vi "ActorDatabase-PerformInsertInstruction.vi"(7 "Payload From Actor":string, 8 "error in (no error)":errorcluster, 11 "Database-Actor in":refnum<class "PartCertDatabase-Actor.lvclass">) -> (0 "error out":errorcluster, 3 "Database-Actor out":refnum<class "PartCertDatabase-Actor.lvclass">)   [LabVIEW 2013, in "PartCertDatabase-Actor.lvclass"]
uses:
  PartCertDatabase-Actor.lvclass
  PartCertDatabase-Actor.lvclass/PartCertDatabase-Actor.ctl
  Reuse Library/Database API/PartCertDatabase-API.lvclass
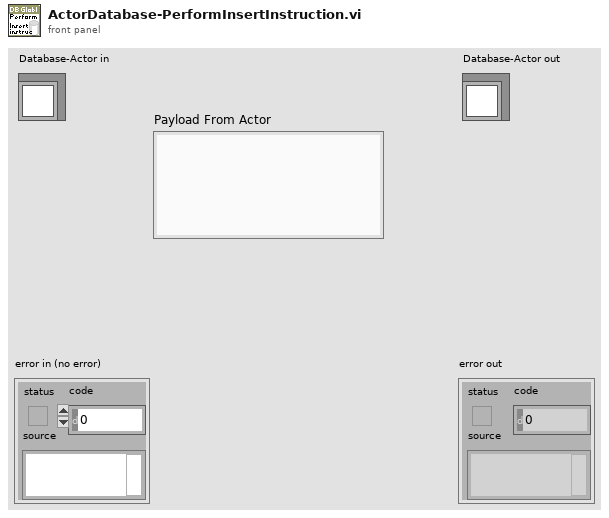
[diagram p1: front panel]
types:
  T1 = cluster{"Table":string, "SQL Statement":string, "Update All":bool, "Payload":string, "Reply Command":string, "Type Of Insertion":i32}
  T2 = cluster{"Manufacturing-Part Number":string, "Step Number":string, "Label Instructions":string, "Path for Picture Label":path, "Path for Picture Label 2":path, "Path for Picture Label 3":path, "Path for Picture Label 4":path, "Path for Picture Label 5":path, "Path for Picture Label 6":path, "Path for Picture Label 7":path, "General Instruction Name":string}[]
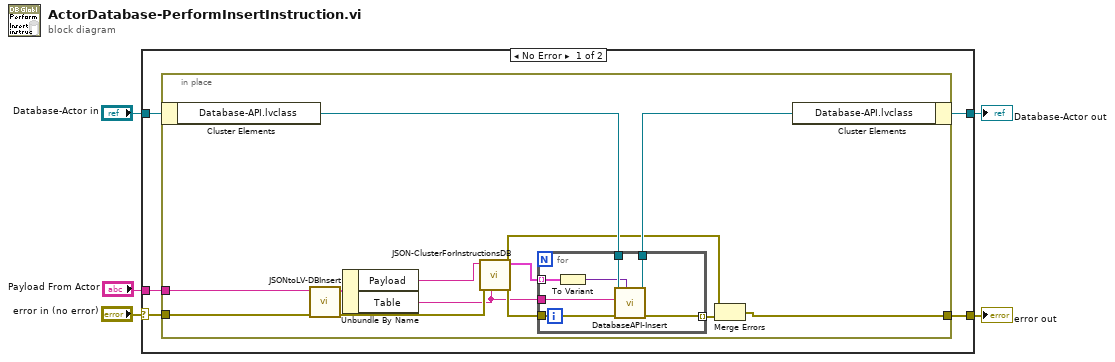
[diagram p0: block diagram]
diagram:
  n1 = case shown="No Error" "error in (no error)" {
    selector: "error in (no error)" -> [w10 w31]
    tunnel: [w9 w31] -> w4
    tunnel: [w7 w30] -> w2
    tunnel: "Database-Actor in" -> [w8 w30]
    tunnel: "Payload From Actor" -> [w6 _]
    frame No Error {
      n2 = in-place {
        in-place-border: w10 -> [w20]
        in-place-border: [w13] -> w9
        in-place-border: w6 -> [w11]
        n3 = in-place-cluster #1(w8) -> ("Database-API.lvclass"=w22:refnum<class "PartCertDatabase-API.lvclass">)
        n4 = call "JSONtoLV-DBInsert.vi"("error in"=w20, "Output JSON Object"=w11) -> ("error out"=w17:errorcluster, "value"=w19:T1)  [unwired: 8 in]
        n5 = Unbundle By Name(w19) -> ("Payload"=w18:string, "Table"=w12:string)
        n6 = call "JSON-ClusterForInstructionsDB.vi"("Table"=w12, "error in (no error)"=w17, "Payload"=w18) -> ("error out"=w14:errorcluster, "Cluster Out"=w16:T2)  [unwired: 7 in]
        n7 = for {
          tunnel: w22 -> [w29]
          tunnel: [w28] -> w21
          tunnel: w12 -> [w27]
          tunnel: w14 -> [w26]
          tunnel: [w25] -> w15 mode=indexing
          tunnel: w16 -> [w24] mode=indexing
          n8 = To Variant(anything=w24) -> (Variant=w23:variant)
          n9 = call "DatabaseAPI-Insert.vi"("Cluster Data for DB"=w23, "error in (no error)"=w26, "Table"=w27, "Database-API in"=w29) -> ("error out"=w25:errorcluster, "Database-API out"=w28:refnum<class "PartCertDatabase-API.lvclass">)  [unwired: 6 in]
        }
        n10 = Merge Errors(w14, w15) -> (w13:errorcluster)
        n11 = in-place-cluster #1("Database-API.lvclass"=w21) -> (w7:refnum<class "PartCertDatabase-Actor.lvclass">)
      }
    }
    frame Error {
    }
  }
  "error out" <- w4
  "Database-Actor out" <- w2
